vi "ParseAllWeeksFromDisk.vi"(11 "RootPath":path=path "C:/data/comics/weeklies") -> (0 "error out":errorcluster, 3 "AllComicURLs":string[](array[string]))   [LabVIEW 2022 SP3]
uses:
  <vilib>/Utility/file.llb/Write Delimited Spreadsheet (string).vi
panel:
  out "Total Count":i32
  out "CurrentFile":string
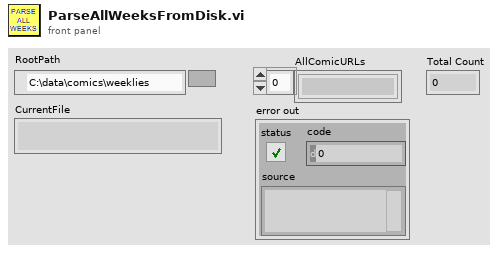
[diagram p1: front panel]
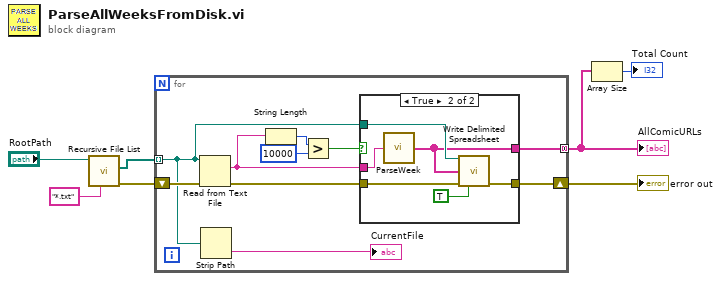
[diagram p0: block diagram]
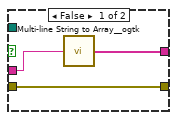
[diagram p2: hidden frame]
diagram:
  n1 = call <vilib>:"Recursive File List.vi"("pattern"="*.txt", "Folder Path"="RootPath") -> ("error out"=w4:errorcluster, "All Files in Dir"=w5:path[])  [unwired: 5 in, 3 out]
  n2 = for {
    tunnel: w5 -> [w15] mode=indexing
    shift-right: [w12] -> w3
    shift-left: w4 -> [w17]
    tunnel: [w14] -> w2 mode=concatenating
    n3 = Read from Text File(file (use dialog)=w15, error in=w17) -> (text=w11:string, error out=w13:errorcluster)  [unwired: 2 in, 2 out]
    n4 = Strip Path(path=w15) -> (name=→"CurrentFile":string)  [unwired: 1 out]
    n5 = String Length(string=w11) -> (length=w10:i32)
    n6 = Greater?(x=w10, y=10000) -> (0:w8:bool)
    n7 = case shown="True" w8 {
      tunnel: w15 -> [_ w26]
      tunnel: [w19 w25] -> w14
      tunnel: w13 -> [w18 w23]
      tunnel: [w18 w22] -> w12
      tunnel: w11 -> [w20 w21]
      frame False {
        n8 = call <userlib>:"Multi-line String to Array__ogtk.vi"("string"=w20) -> ("lines"=w19:string[])
      }
      frame True {
        n9 = call "ParseWeek.vi"("HTML  Body"=w21) -> ("ComicURLs"=w25:string[])
        n10 = call-poly <vilib>:"Write Delimited Spreadsheet.vi"("file path (dialog if empty)"=w26, "1D data"=w25, "error in (no error)"=w23, "transpose? (no:F)"=TRUE) -> ("error out"=w22:errorcluster)  [unwired: 10 in, 1 out]
      }
    }
  }
  "AllComicURLs" <- w2
  "error out" <- w3
  n11 = Array Size(array=w2) -> (size(s)=→"Total Count":i32)
